vi "Send Set State.vi"(7 "Message Priority (Normal)":T2=enum."Normal", 8 "error in (no error)":errorcluster, 10 "State":T1, 11 "Message Enqueuer":refnum<class "Message Enqueuer.lvclass">) -> (0 "error out":errorcluster, 3 "Message Enqueuer out":refnum<class "Message Enqueuer.lvclass">)   [LabVIEW 2019, in "Elevator Controller.lvlib" / "Set State Msg.lvclass"]
doc: "This VI sends the message to an actor."
uses:
  Set State Msg.lvclass
  <vilib>/ActorFramework/Message Enqueuer/Message Enqueuer.lvclass
  <vilib>/ActorFramework/Message Enqueuer/Message Priority.ctl
  Elevator Controller/State -Enum.ctl
  C:/Program Files (x86)/National Instruments/LabVIEW 2019/vi.lib/ActorFramework/Message/Message.lvclass
  Set State Msg.lvclass/Set State Msg.ctl
  <vilib>/ActorFramework/Message Enqueuer/Message Enqueuer.lvclass/Message Enqueuer.ctl
  <vilib>/ActorFramework/Message Priority Queue/Priority Enqueue.vi
  Elevator Controller/Elevator Controller.lvclass
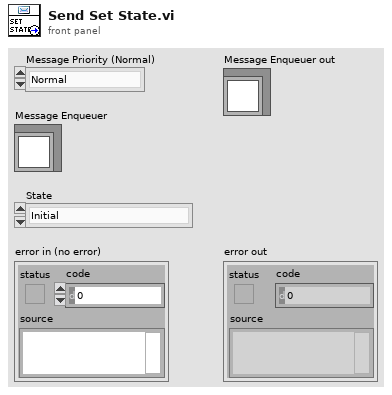
[diagram p1: front panel]
types:
  T1 = typedef "Elevator Controller.lvlib/Elevator Controller.lvclass/State -Enum.ctl" = enum16{"Initial", "Wait for First Request", "Start and Move", "Analysis", "Continue Travel", "Stop at Floor", "Open and Close Door Sequence", "No request Remaining", "Emergency Call", "Terminate Process"}
  T2 = typedef "Actor Framework.lvlib/Message Enqueuer.lvclass/Message Priority.ctl" = enum16{"Low", "Normal", "High"}
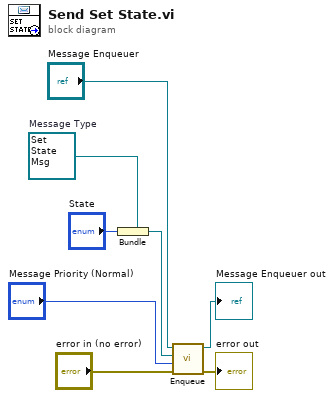
[diagram p0: block diagram]
diagram:
  w5 = refnum<class "Set State Msg.lvclass"> refnum  # Message Type
  n1 = Bundle(cluster=w5, "State") -> (w4:refnum<class "Set State Msg.lvclass">)
  n2 = call <vilib>:"Enqueue.vi"("error in (no error)"="error in (no error)", "Message Priority (Normal)"="Message Priority (Normal)", "Message"=w4, "Message Enqueuer in"="Message Enqueuer") -> ("error out"=→"error out":errorcluster, "Message Enqueuer out"=→"Message Enqueuer out":refnum<class "Message Enqueuer.lvclass">)  [unwired: 6 in]
